vi "一体站流程平行样自动启动.vi"(11 "参数":T1) -> ()   [LabVIEW 2016, in "质控单元.lvlib"]
panel:
  out "枚举":enum16{"初始化", "采配水启动", "等待", "配水", "排水", "结束"}(ring)
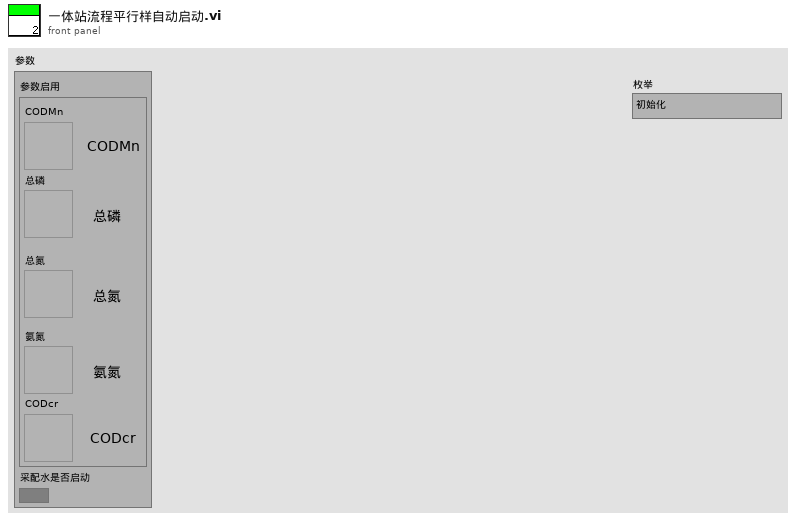
[diagram p1: front panel]
types:
  T1 = cluster{"参数启用":cluster{"CODMn":bool, "总磷":bool, "总氮":bool, "氨氮":bool, "CODcr":bool}, "采配水是否启动":bool}
  T2 = cluster{"命令":string, cluster{"starting address":u16, "holding register value":u16}}
  T3 = typedef "质控单元.lvlib/平行样测试流程.ctl" = enum16{"待机", "第一次水样测试启动", "第一次水样测试中", "第二次水样测试启动", "第二次水样测试中", "存储平行样测试数据", "结束"}
  T4 = cluster{"站号":u16, "量程切换":enum32{"H", "L", "AUTO"}, "控制命令":enum16{"启动测量", "标样核查", "零点核查", "跨度核查", "空白测试", "平行样测试", "加标回收", "空白校准", "标样校准", "初始化（清洗）", "停止测试", "仪器重启", "校时", "模式设置", "测量间隔设置"}, "模式设置":enum16{"待机", "连续模式", "周期模式", "定点模式", "受控模式", "手动模式"}, "测量间隔":u16}
  T5 = cluster{"时间标识":timestamp, "设备":string, "日志信息":string}
  T6 = enum16{"空闲", "水样测试", "标样核查", "零点核查", "跨度核查", "空白测试", "平行样测试", "加标回收", "空白校准", "标样校准", "初始化（清洗）"}
  T7 = cluster{"测量模式":enum16{"水样测量", "标样核查", "零点核查", "跨度核查", "空白测试", "加标回收", "平行样", "校零", "校标"}}
  T8 = cluster{"时间标识":timestamp, "设备":string, "日志信息":string, "流程参数":string}
  T9 = cluster{"R0":i16, "R1":i16, "R2":i16, "R3":i16, "R4":i16, "R5":i16, "R6":i16, "R7":i16, "R8":i16, "R9":i16, "R10":i16, "R11":i16, "R12":i16, "R13":i16, "R14":i16, "R15":i16, "R16":i16, "R17":i16, "R18":i16, "R19":i16, "R20":i16, "R21":i16, "R22":i16, "R23":i16, "R24":i16, "R25":i16, "R26":i16, "R27":i16, "R28":i16, "R29":i16, "R30":i16, "R31":i16, "R32":i16, "R33":i16, "R34":i16, "R35":i16, "R36":i16, "R37":i16, "R38":i16, "R39":i16, "R40":i16, "R41":i16, "R42":i16, "R43":i16, "R44":i16, "R45":i16, "R46":i16, "R47":i16, "R48":i16, "R49":i16, "R50":i16, "R51":i16, "R52":i16, "R53":i16, "R54":i16, "R55":i16, "R56":i16}
  T10 = cluster{"系统时间":timestamp, "工作状态":enum16{"空闲", "水样测试", "标样核查", "零点核查", "跨度核查", "空白测试", "平行样测试", "加标回收", "空白校准", "标样校准", "初始化（清洗）"}, "测量模式":enum16{"待机", "连续模式", "周期模式", "定点模式", "受控模式", "手动模式"}, "告警代码":enum16{"无告警", "缺试剂告警", "缺水样告警", "缺蒸馏水告警", "缺标液告警", "仪表漏液告警", "标定异常告警", "超量程告警", "加热异常", "低试剂预警", "超上限告警", "超下限告警", "仪表内部其他异常", "滴定异常告警", "电极异常告警", "量程切换告警", "参数设置告警", "PH电极电位异常", "电导率电极异常", "浊度光度异常", "溶解氧电极异常", "溶解氧光强异常", "温度异常告警", "PH异常告警", "溶解氧异常告警", "电导率异常告警", "浊度异常告警", "叶绿素异常告警", "藻密度异常告警", "蓝绿藻异常告警", "ORP异常告警", "氨氮异常告警", "清洁刷异常告警", "SD卡异常告警", "蓝牙异常告警", "Wifi异常告警", "流程异常告警"}, "故障代码":enum16{"无故障", "电机故障", "温度故障", "通讯故障", "滴定故障"}, "日志代码":u16, "软件版本":u16, "F0":sgl, "F1":sgl, "F2":sgl, "F3":sgl, "T":sgl, "H":sgl, "id":u16, "flowid":u16, "量程":u16, "总磷控温温度1":sgl, "营养盐控温温度2":sgl, "ADC":sgl}
  T11 = cluster{"因子编码":u32, "单位":u16, "标样参考值":sgl, "水样数据时间":timestamp, "水样实测值":sgl, "水样数据标识":string, "标样数据时间":timestamp, "标样实测值":sgl, "标样数据标识":string, "空白数据时间":timestamp, "空白实测值":sgl, "空白数据标识":string, "零点核查数据时间":timestamp, "零点核查实测值":sgl, "零点核查数据标识":string, "跨度核查数据时间":timestamp, "跨度核查实测值":sgl, "跨度核查数据标识":string, "加标回收数据时间":timestamp, "加标回收实测值":sgl, "加标回收数据标识":string, "平行样数据时间":timestamp, "平行样实测值":sgl, "平行样数据标识":string}
  T12 = cluster{"时间标识":timestamp, "参数":string, "数据类型":string, "第一次水样浓度值":sgl, "第二次水样测试时间":timestamp, "第二次水样浓度值":sgl}
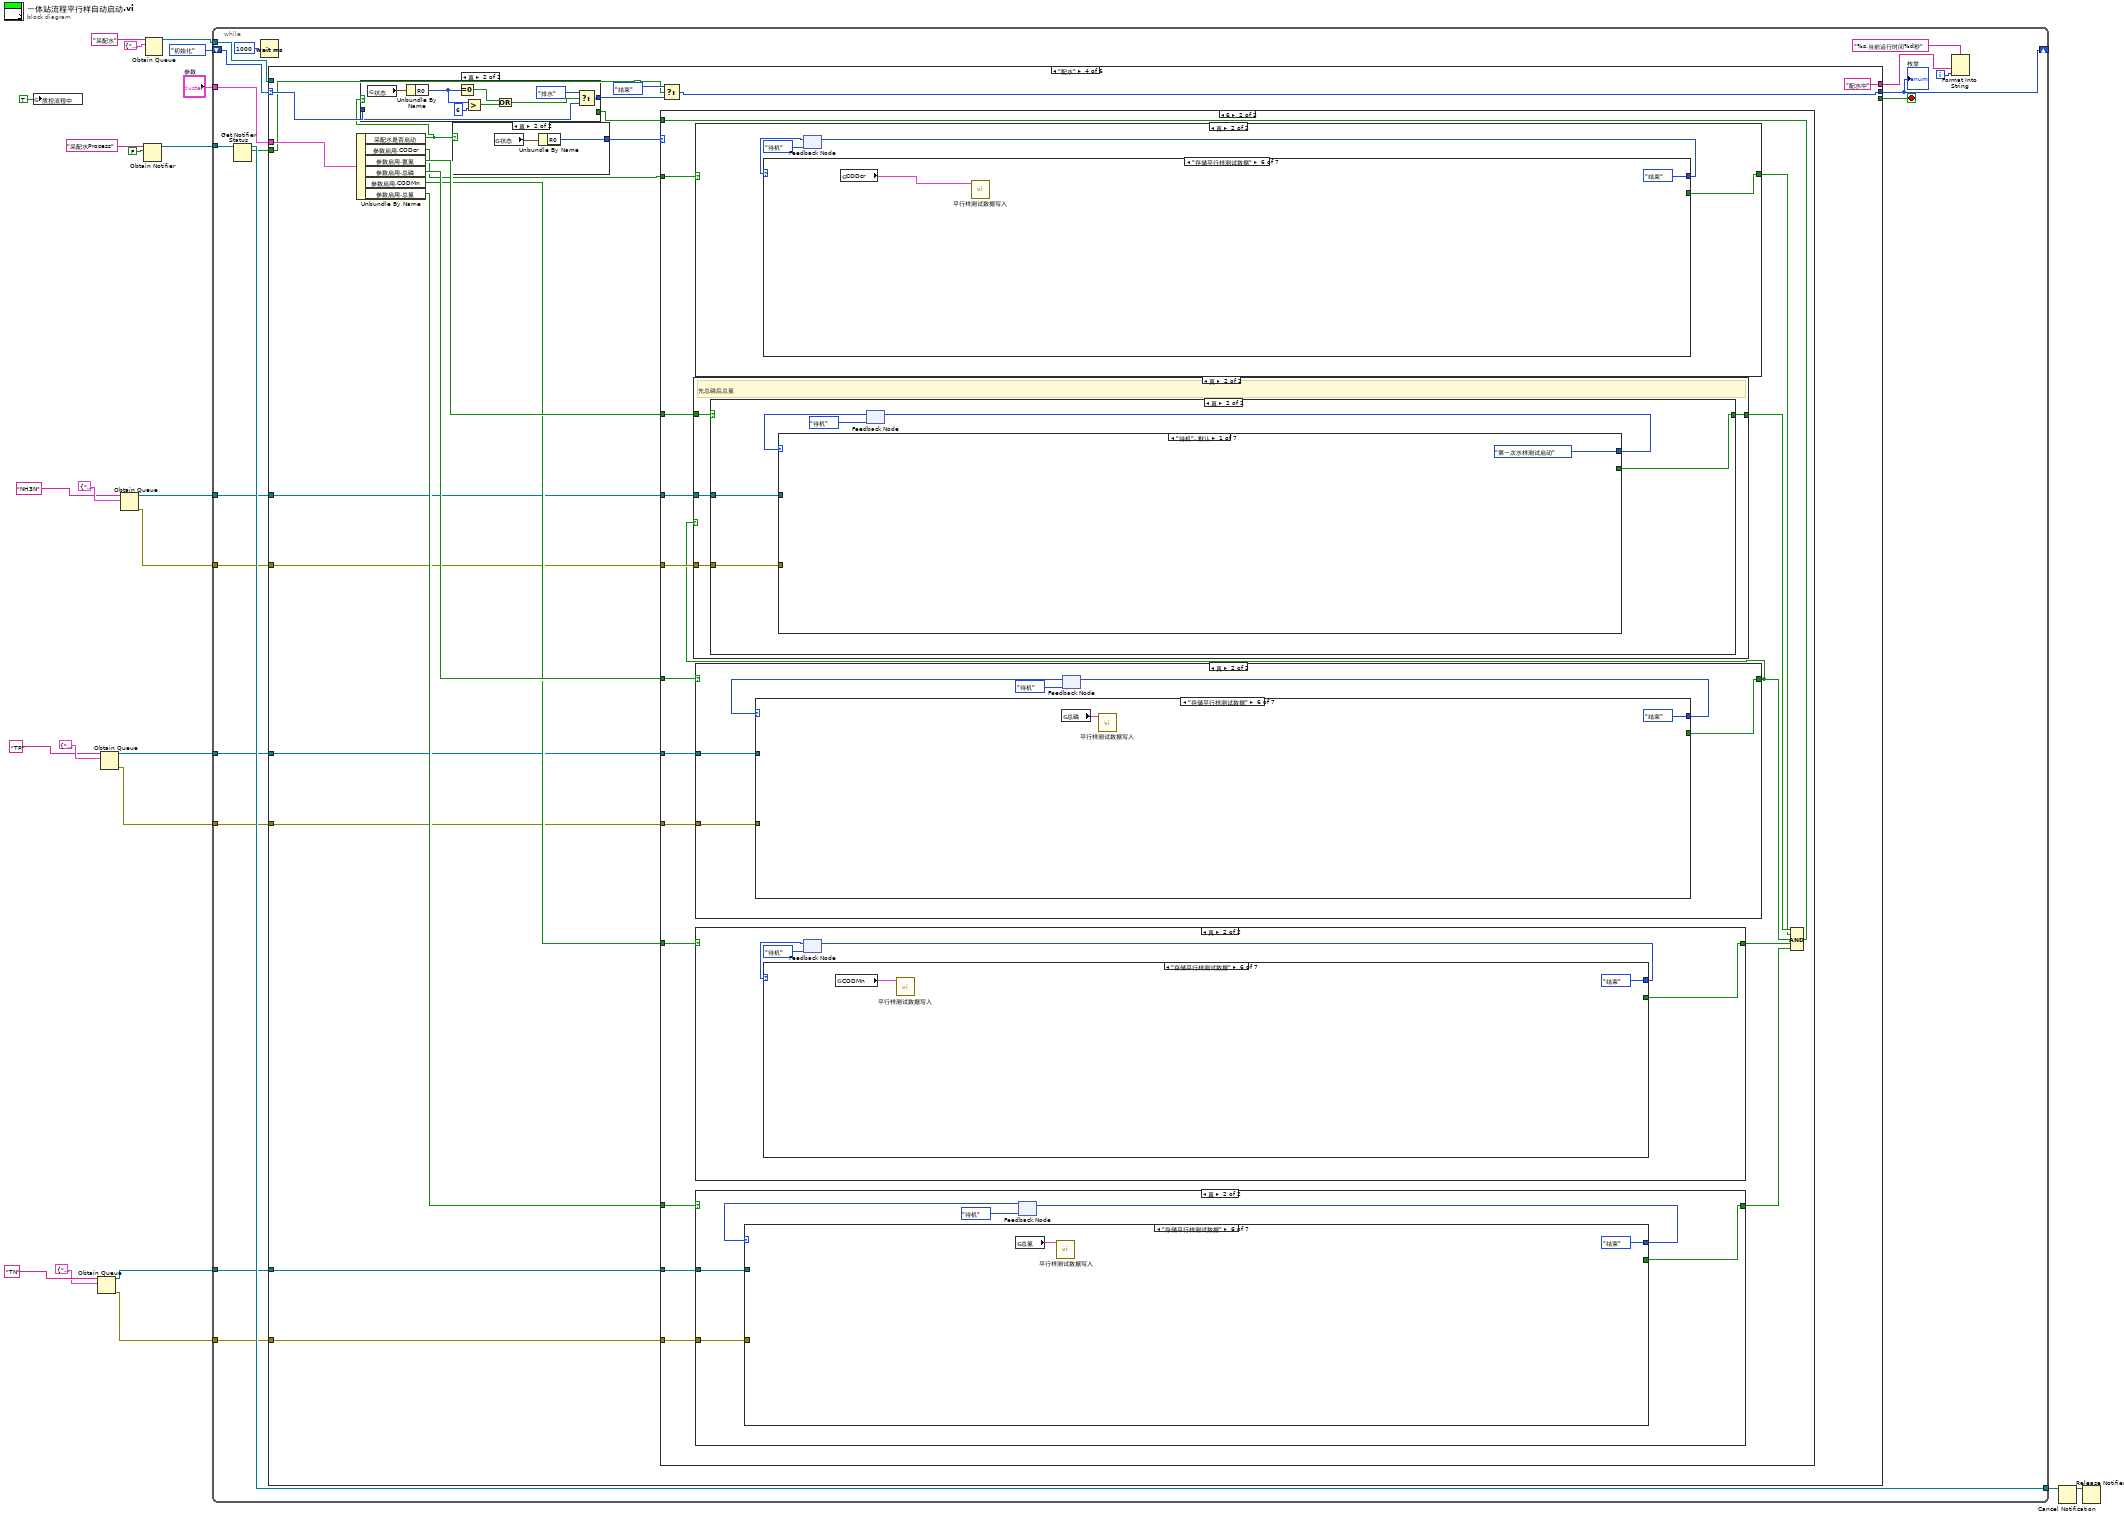
[diagram p0: block diagram]
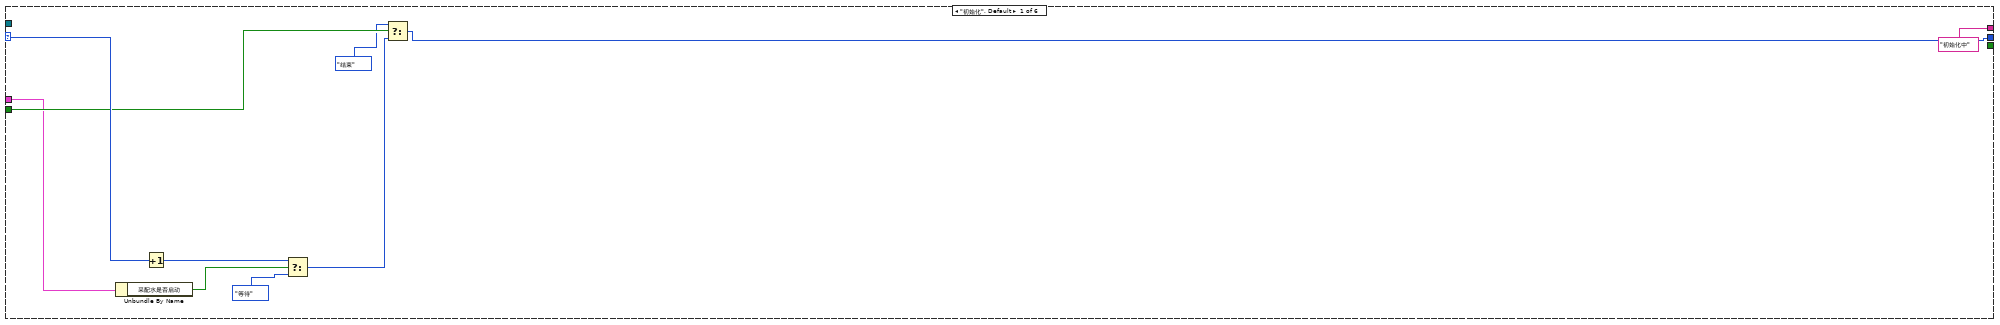
[diagram p2: hidden frame]
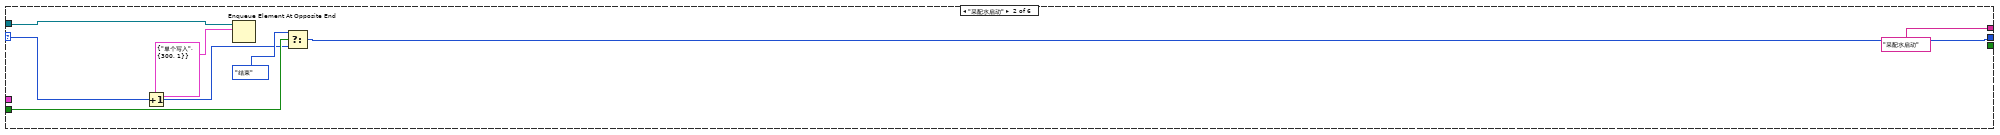
[diagram p3: hidden frame]
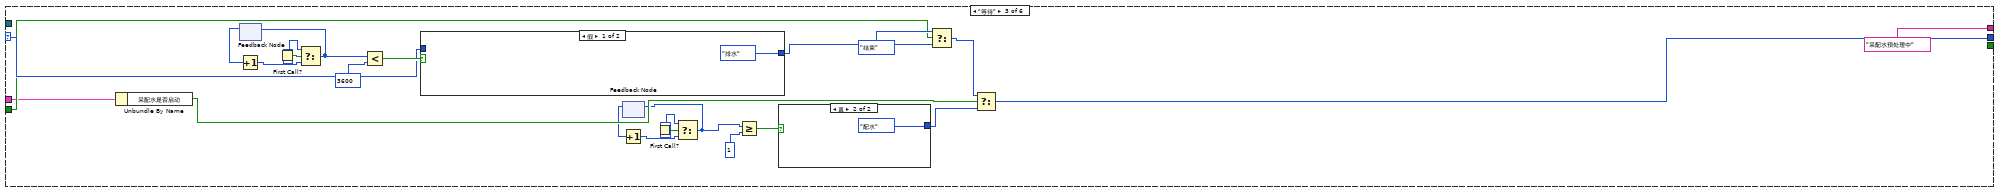
[diagram p4: hidden frame]
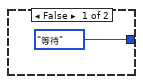
[diagram p5: hidden frame]
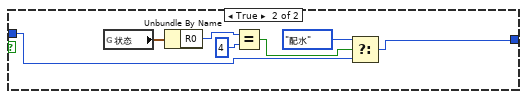
[diagram p6: hidden frame]
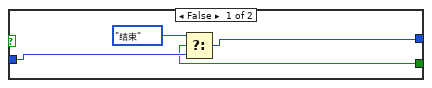
[diagram p7: hidden frame]
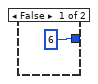
[diagram p8: hidden frame]
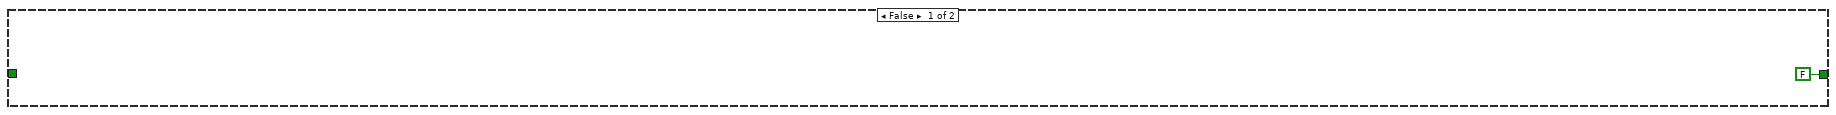
[diagram p10: hidden frame]
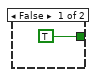
[diagram p11: hidden frame]
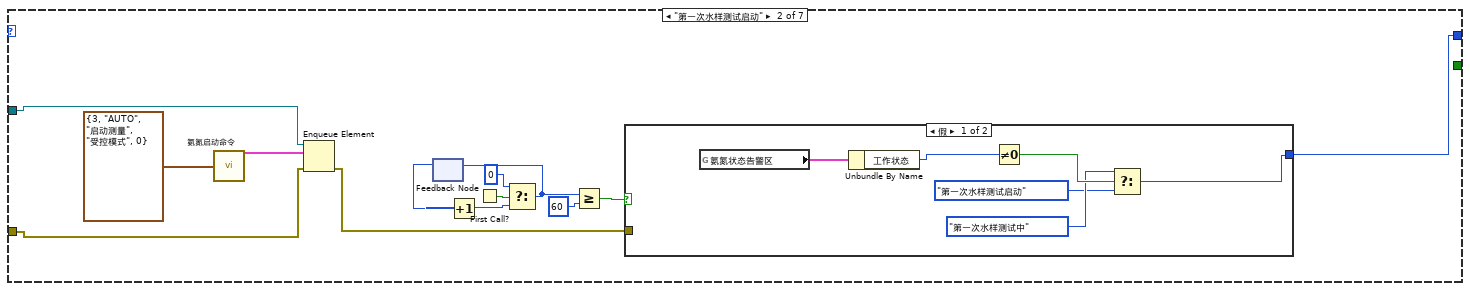
[diagram p12: hidden frame]
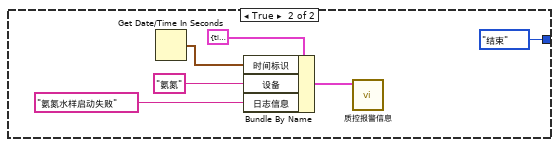
[diagram p13: hidden frame]
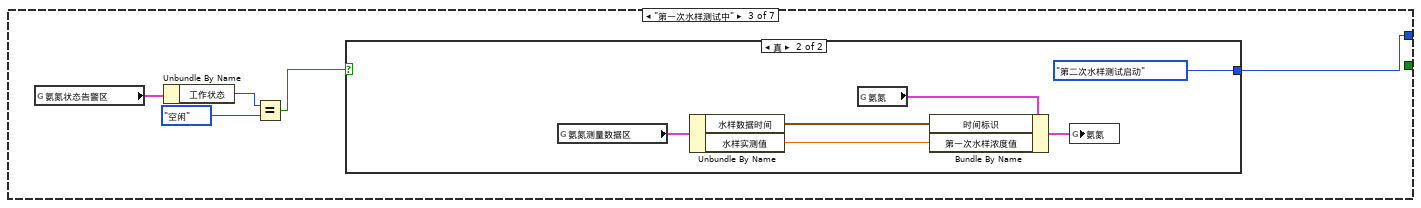
[diagram p14: hidden frame]
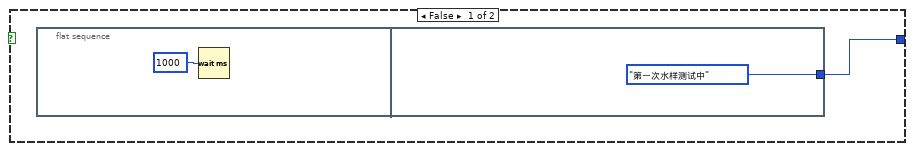
[diagram p15: hidden frame]
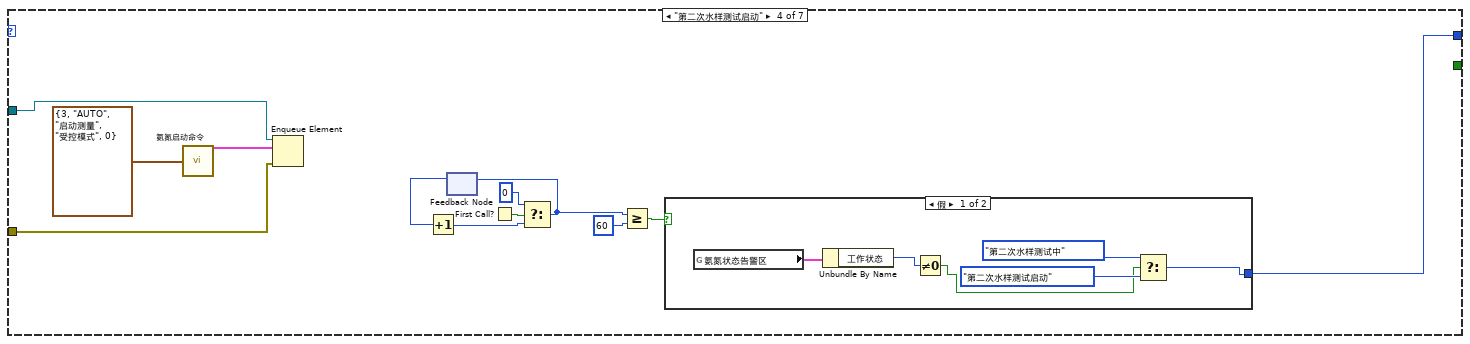
[diagram p16: hidden frame]
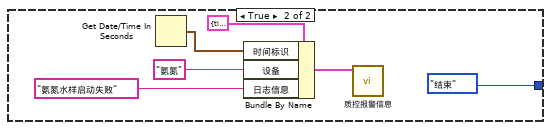
[diagram p17: hidden frame]
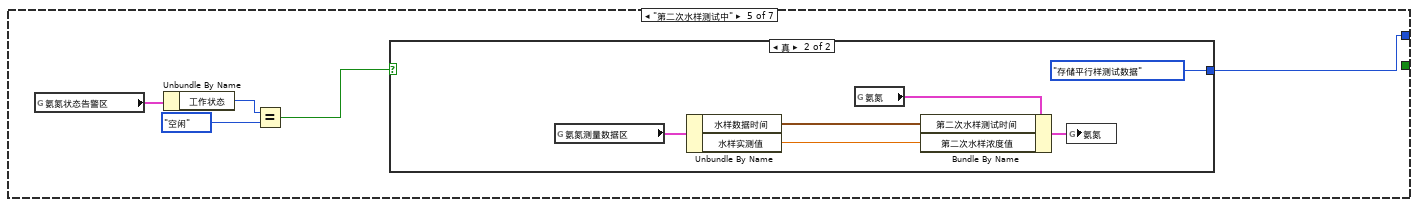
[diagram p18: hidden frame]
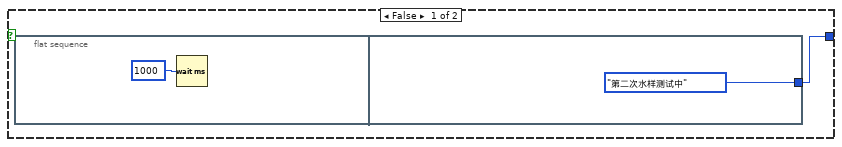
[diagram p19: hidden frame]
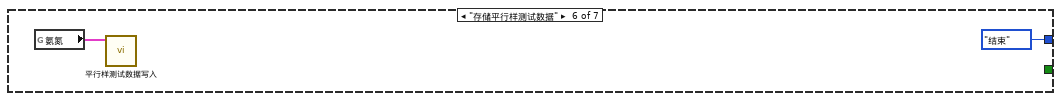
[diagram p20: hidden frame]
diagram:
  n1 = global write "质控测完标志全局 1.vi" "质控流程中"(TRUE ("质控流程中")) -> ()
  n2 = Obtain Queue(name (unnamed)="TN" ("名称（未命名）"), element data type=cluster{"命令":string, "data":variant} {"命令"="", "data"=variant}) -> (queue out=w3:refnum<queue>, error out=w2:errorcluster)  [unwired: 3 in, 1 out]
  n3 = Obtain Queue(name (unnamed)="TP" ("名称（未命名）"), element data type=cluster{"命令":string, "data":variant} {"命令"="", "data"=variant}) -> (queue out=w5:refnum<queue>, error out=w4:errorcluster)  [unwired: 3 in, 1 out]
  n4 = Obtain Queue(name (unnamed)="NH3N" ("名称（未命名）"), element data type=cluster{"命令":string, "data":variant} {"命令"="", "data"=variant}) -> (queue out=w7:refnum<queue>, error out=w6:errorcluster)  [unwired: 3 in, 1 out]
  n5 = Obtain Notifier(name (unnamed)="采配水Process" ("名称（未命名）"), notification data type=FALSE) -> (notifier out=w16:refnum<notifier>)  [unwired: 2 in, 2 out]
  n6 = Obtain Queue(name (unnamed)="采配水" ("名称（未命名）"), element data type=cluster{"命令":string, "数据":variant} {"命令"="", "数据"=variant}) -> (queue out=w21:refnum<queue>)  [unwired: 3 in, 2 out]
  n7 = while {
    tunnel: w21 -> [w41]
    shift-right: [w39] -> _
    shift-left: enum16{"初始化", "采配水启动", "等待", "配水", "排水", "结束"}."初始化" ("枚举") -> [w40]
    tunnel: "参数" -> [w37]
    tunnel: w16 -> [w36]
    tunnel: [w35] -> w15
    tunnel: w7 -> [w30]
    tunnel: w6 -> [w29]
    tunnel: w5 -> [w28]
    tunnel: w4 -> [w27]
    tunnel: w3 -> [w26]
    tunnel: w2 -> [w25]
    i -> [w32]
    stop <- w24 stop-if-true
    n8 = Get Notifier Status(notifier=w36) -> (notifier out=w35:refnum<notifier>, current notification=w31:bool)  [unwired: 1 in, 3 out]
    n9 = Wait (ms)(milliseconds to wait=u32 1000 ("等待时间（毫秒）")) -> ()  [unwired: 1 out]
    n10 = case shown="\"配水\"" w40 {
      selector: w40 -> [w51 w57 w81 w114 w596 w603]
      tunnel: w41 -> [_ w58 _ _ w597 _]
      tunnel: [w48 w52 w60 w111 w591 w602] -> w39
      tunnel: [_ _ _ _ _ TRUE] -> w24
      tunnel: w37 -> [w46 _ w71 w107 _ _]
      tunnel: ["初始化中" ("输入 1") "采配水启动" ("输入 1") "采配水预处理中" ("输入 1") "配水中" ("输入 1") "排水中" ("输入 1") "结束" ("输入 1")] -> w33
      tunnel: w31 -> [w49 w54 w73 w95 w593 _]
      tunnel: w30 -> [_ _ _ w102 _ _]
      tunnel: w29 -> [_ _ _ w101 _ _]
      tunnel: w28 -> [_ _ _ w100 _ _]
      tunnel: w27 -> [_ _ _ w99 _ _]
      tunnel: w26 -> [_ _ _ w98 _ _]
      tunnel: w25 -> [_ _ _ w97 _ _]
      frame "初始化", Default {
        n11 = Unbundle By Name(w46) -> ("采配水是否启动"=w45:bool)
        n12 = Increment(x=w51) -> (x+1=w44:enum16{"初始化", "采配水启动", "等待", "配水", "排水", "结束"})
        n13 = Select(t=w44, s=w45, f=enum16{"初始化", "采配水启动", "等待", "配水", "排水", "结束"}."等待") -> (s? t:f=w43:enum16{"初始化", "采配水启动", "等待", "配水", "排水", "结束"})
        n14 = Select(t=enum16{"初始化", "采配水启动", "等待", "配水", "排水", "结束"}."结束", s=w49, f=w43) -> (s? t:f=w48:enum16{"初始化", "采配水启动", "等待", "配水", "排水", "结束"})
      }
      frame "采配水启动" {
        n15 = Increment(x=w57) -> (x+1=w53:enum16{"初始化", "采配水启动", "等待", "配水", "排水", "结束"})
        n16 = Enqueue Element At Opposite End(queue=w58, element=T2 {"命令"="单个写入", {"starting address"=300, "holding register value"=1}} ("元素")) -> ()  [unwired: 2 in, 3 out]
        n17 = Select(t=enum16{"初始化", "采配水启动", "等待", "配水", "排水", "结束"}."结束", s=w54, f=w53) -> (s? t:f=w52:enum16{"初始化", "采配水启动", "等待", "配水", "排水", "结束"})
      }
      frame "等待" {
        n18 = Unbundle By Name(w71) -> ("采配水是否启动"=w70:bool)
        n19 = feedback #1() -> (w78:i32)  [unwired: 1 in]
        n20 = Increment(x=w78) -> (x+1=w77:i32)
        n21 = First Call?() -> (First Call?: T/F=w79:bool)
        n22 = Select(t=0, s=w79, f=w77) -> (s? t:f=w76:i32)
        n23 = feedback-in #1(w76) -> ()
        n24 = Less?(x=w76, y=3600) -> (x < y?=w82:bool)
        n25 = case shown="假" w82 {
          tunnel: w81 -> [_ w88]
          tunnel: [enum16{"初始化", "采配水启动", "等待", "配水", "排水", "结束"}."排水" ("枚举") w87] -> w72
          frame False {
          }
          frame True {
            n26 = global read "与采配水交互全局.vi" "状态"() -> (w93:T9)
            n27 = Unbundle By Name(w93) -> ("R0"=w92:i16)
            n28 = Equal?(x=w92, y=i16 4) -> (x = y?=w90:bool)
            n29 = Select(t=enum16{"初始化", "采配水启动", "等待", "配水", "排水", "结束"}."配水" ("枚举"), s=w90, f=w88) -> (s? t:f=w87:enum16{"初始化", "采配水启动", "等待", "配水", "排水", "结束"})
          }
        }
        n30 = feedback #2() -> (w66:i32)  [unwired: 1 in]
        n31 = Increment(x=w66) -> (x+1=w67:i32)
        n32 = First Call?() -> (First Call?: T/F=w65:bool)
        n33 = Select(t=0, s=w65, f=w67) -> (s? t:f=w68:i32)
        n34 = feedback-in #2(w68) -> ()
        n35 = Greater Or Equal?(x=w68, y=1) -> (x >= y?=w62:bool)
        n36 = case shown="真" w62 {
          tunnel: [enum16{"初始化", "采配水启动", "等待", "配水", "排水", "结束"}."等待" ("t") enum16{"初始化", "采配水启动", "等待", "配水", "排水", "结束"}."配水" ("t")] -> w61
          frame False {
          }
          frame True {
          }
        }
        n37 = Select(t=enum16{"初始化", "采配水启动", "等待", "配水", "排水", "结束"}."结束", s=w73, f=w72) -> (s? t:f=w69:enum16{"初始化", "采配水启动", "等待", "配水", "排水", "结束"})
        n38 = Select(t=w69, s=w70, f=w61) -> (s? t:f=w60:enum16{"初始化", "采配水启动", "等待", "配水", "排水", "结束"})
      }
      frame "配水" {
        n39 = Unbundle By Name(w107) -> ("采配水是否启动"=w96:bool, "参数启用.CODcr"=w106:bool, "参数启用.氨氮"=w110:bool, "参数启用.总磷"=w109:bool, "参数启用.CODMn"=w108:bool, "参数启用.总氮"=w105:bool)
        n40 = case shown="真" w96 {
          tunnel: [i16 6 ("R0") w129] -> w104
          frame False {
          }
          frame True {
            n41 = global read "与采配水交互全局.vi" "状态"() -> (w130:T9)
            n42 = Unbundle By Name(w130) -> ("R0"=w129:i16)
          }
        }
        n43 = case shown="6" w104 {
          tunnel: w110 -> [_ w147]
          tunnel: w109 -> [_ w146]
          tunnel: w108 -> [_ w144]
          tunnel: w106 -> [_ w143]
          tunnel: w105 -> [_ w140]
          tunnel: w102 -> [_ w138]
          tunnel: w101 -> [_ w137]
          tunnel: w100 -> [_ w136]
          tunnel: w99 -> [_ w135]
          tunnel: w98 -> [_ w134]
          tunnel: w97 -> [_ w133]
          tunnel: [_ w132] -> w94
          frame 0, Default {
          }
          frame 6 {
            n44 = case shown="真" w143 {
              tunnel: [TRUE w408] -> w142
              frame False {
              }
              frame True {
                n45 = feedback #3(平行样测试流程."待机") -> (w410:T3)
                n46 = case shown="\"存储平行样测试数据\"" w410 {
                  tunnel: [平行样测试流程."第一次水样测试启动" w422 w444 w464 w486 平行样测试流程."结束" 平行样测试流程."结束"] -> w409
                  tunnel: [_ _ _ _ _ _ TRUE] -> w408
                  frame "待机", Default {
                  }
                  frame "第一次水样测试启动" {
                    n47 = call "CODCr启动命令 (子VI).vi"("启动测量模式"=T7 {"测量模式"=enum."水样测量"}) -> ("错误输出"=w412:errorcluster)  [unwired: 10 in]
                    n48 = First Call?() -> (First Call?: T/F=w414:bool)
                    n49 = case shown="真" w414 {
                      frame False {
                      }
                      frame True {
                        n50 = Get Date/Time In Seconds() -> (seconds since 1Jan1904=w425:timestamp)
                        n51 = Bundle By Name(cluster=T8 {"时间标识"=timestamp(0 s since 1904-01-01), "设备"="", "日志信息"="", "流程参数"=""} ("data in"), "时间标识"=w425, "设备"="CODCr", "日志信息"="-->>CODCr启动水样") -> (w426:T8)
                        n52 = call "质控日志存储 (子VI).vi"("data in"=w426) -> ()  [unwired: 11 in]
                      }
                    }
                    n53 = feedback #4() -> (w418:i32)  [unwired: 1 in]
                    n54 = Increment(x=w418) -> (x+1=w419:i32)
                    n55 = First Call?() -> (First Call?: T/F=w417:bool)
                    n56 = Select(t=0, s=w417, f=w419) -> (s? t:f=w420:i32)
                    n57 = feedback-in #4(w420) -> ()
                    n58 = Greater Or Equal?(x=w420, y=60) -> (x >= y?=w415:bool)
                    n59 = case shown="假" w415 {
                      tunnel: [w432 平行样测试流程."结束"] -> w422
                      tunnel: w412 -> [_ _]
                      frame False {
                        n60 = global read "与CODCr交互全局.vi" "CODCr状态告警区"() -> (w429:T10)
                        n61 = Unbundle By Name(w429) -> ("工作状态"=w428:T6)
                        n62 = Not Equal To 0?(x=w428) -> (x != 0?=w433:bool)
                        n63 = Select(t=平行样测试流程."第一次水样测试中", s=w433, f=平行样测试流程."第一次水样测试启动") -> (s? t:f=w432:T3)
                      }
                      frame True {
                        n64 = Get Date/Time In Seconds() -> (seconds since 1Jan1904=w436:timestamp)
                        n65 = Bundle By Name(cluster=T5 {"时间标识"=timestamp(0 s since 1904-01-01), "设备"="", "日志信息"=""} ("data in"), "时间标识"=w436, "设备"="CODCr", "日志信息"="CODCr水样启动失败") -> (w434:T5)
                        n66 = call "质控报警信息.vi"("data in"=w434) -> ()  [unwired: 11 in]
                      }
                    }
                  }
                  frame "第一次水样测试中" {
                    n67 = global read "与CODCr交互全局.vi" "CODCr状态告警区"() -> (w443:T10)
                    n68 = Unbundle By Name(w443) -> ("工作状态"=w440:T6)
                    n69 = Equal?(x=w440, y=T6."空闲" ("工作状态")) -> (x = y?=w442:bool)
                    n70 = case shown="真" w442 {
                      tunnel: [w445 平行样测试流程."第二次水样测试启动"] -> w444
                      frame False {
                        n71 = flat-sequence {
                          tunnel: [平行样测试流程."第一次水样测试中"] -> w445
                          frame #0 {
                            n72 = Wait (ms)(milliseconds to wait=u32 1000 ("等待时间（毫秒）")) -> ()  [unwired: 1 out]
                          }
                          frame #1 {
                          }
                        }
                      }
                      frame True {
                        n73 = global read "与CODCr交互全局.vi" "CODCr测量数据区"() -> (w450:T11)
                        n74 = Unbundle By Name(w450) -> ("水样数据时间"=w449:timestamp, "水样实测值"=w448:sgl)
                        n75 = global read "平行样测试全局变量.vi" "CODcr"() -> (w452:T12)
                        n76 = Bundle By Name(cluster=w452, "时间标识"=w449, "第一次水样浓度值"=w448) -> (w451:T12)
                        n77 = global write "平行样测试全局变量.vi" "CODcr"(w451) -> ()
                      }
                    }
                  }
                  frame "第二次水样测试启动" {
                    n78 = call "CODCr启动命令 (子VI).vi"("启动测量模式"=T7 {"测量模式"=enum."水样测量"}) -> ("错误输出"=w454:errorcluster)  [unwired: 10 in]
                    n79 = First Call?() -> (First Call?: T/F=w456:bool)
                    n80 = case shown="真" w456 {
                      frame False {
                      }
                      frame True {
                        n81 = Get Date/Time In Seconds() -> (seconds since 1Jan1904=w467:timestamp)
                        n82 = Bundle By Name(cluster=T8 {"时间标识"=timestamp(0 s since 1904-01-01), "设备"="", "日志信息"="", "流程参数"=""} ("data in"), "时间标识"=w467, "设备"="CODCr", "日志信息"="-->>CODCr启动水样") -> (w468:T8)
                        n83 = call "质控日志存储 (子VI).vi"("data in"=w468) -> ()  [unwired: 11 in]
                      }
                    }
                    n84 = First Call?() -> (First Call?: T/F=w459:bool)
                    n85 = feedback #5() -> (w460:i32)  [unwired: 1 in]
                    n86 = Increment(x=w460) -> (x+1=w461:i32)
                    n87 = Select(t=0, s=w459, f=w461) -> (s? t:f=w462:i32)
                    n88 = feedback-in #5(w462) -> ()
                    n89 = Greater Or Equal?(x=w462, y=60) -> (x >= y?=w457:bool)
                    n90 = case shown="假" w457 {
                      tunnel: [w474 平行样测试流程."结束"] -> w464
                      tunnel: w454 -> [_ _]
                      frame False {
                        n91 = global read "与CODCr交互全局.vi" "CODCr状态告警区"() -> (w471:T10)
                        n92 = Unbundle By Name(w471) -> ("工作状态"=w470:T6)
                        n93 = Not Equal To 0?(x=w470) -> (x != 0?=w475:bool)
                        n94 = Select(t=平行样测试流程."第二次水样测试中", s=w475, f=平行样测试流程."第二次水样测试启动") -> (s? t:f=w474:T3)
                      }
                      frame True {
                        n95 = Get Date/Time In Seconds() -> (seconds since 1Jan1904=w478:timestamp)
                        n96 = Bundle By Name(cluster=T5 {"时间标识"=timestamp(0 s since 1904-01-01), "设备"="", "日志信息"=""} ("data in"), "时间标识"=w478, "设备"="CODCr", "日志信息"="CODCr启动失败") -> (w476:T5)
                        n97 = call "质控报警信息.vi"("data in"=w476) -> ()  [unwired: 11 in]
                      }
                    }
                  }
                  frame "第二次水样测试中" {
                    n98 = global read "与CODCr交互全局.vi" "CODCr状态告警区"() -> (w485:T10)
                    n99 = Unbundle By Name(w485) -> ("工作状态"=w482:T6)
                    n100 = Equal?(x=w482, y=T6."空闲" ("工作状态")) -> (x = y?=w484:bool)
                    n101 = case shown="假" w484 {
                      tunnel: [w487 平行样测试流程."存储平行样测试数据"] -> w486
                      frame False {
                        n102 = flat-sequence {
                          tunnel: [平行样测试流程."第二次水样测试中"] -> w487
                          frame #0 {
                            n103 = Wait (ms)(milliseconds to wait=u32 1000 ("等待时间（毫秒）")) -> ()  [unwired: 1 out]
                          }
                          frame #1 {
                          }
                        }
                      }
                      frame True {
                        n104 = global read "与CODCr交互全局.vi" "CODCr测量数据区"() -> (w492:T11)
                        n105 = Unbundle By Name(w492) -> ("水样数据时间"=w491:timestamp, "水样实测值"=w490:sgl)
                        n106 = global read "平行样测试全局变量.vi" "CODcr"() -> (w494:T12)
                        n107 = Bundle By Name(cluster=w494, "第二次水样测试时间"=w491, "第二次水样浓度值"=w490) -> (w493:T12)
                        n108 = global write "平行样测试全局变量.vi" "CODcr"(w493) -> ()
                      }
                    }
                  }
                  frame "存储平行样测试数据" {
                    n109 = global read "平行样测试全局变量.vi" "CODcr"() -> (w496:T12)
                    n110 = call "平行样测试数据写入.vi"("data"=w496) -> ()  [unwired: 10 in, 1 out]
                  }
                  frame "结束" {
                    n111 = First Call?() -> (First Call?: T/F=w499:bool)
                    n112 = case shown="真" w499 {
                      frame False {
                      }
                      frame True {
                        (unwired) "-->>CODCr停止" ("日志信息")
                        (unwired) "CODCr" ("设备")
                        n113 = call "质控日志存储 (子VI).vi"() -> ()  [unwired: 12 in]
                      }
                    }
                  }
                }
                n114 = feedback-in #3(w409) -> ()
              }
            }
            n115 = case shown="真" w146 {
              tunnel: [TRUE w505] -> w131
              tunnel: w136 -> [_ w503]
              tunnel: w135 -> [_ w502]
              frame False {
              }
              frame True {
                n116 = feedback #6(平行样测试流程."待机") -> (w507:T3)
                n117 = case shown="\"存储平行样测试数据\"" w507 {
                  tunnel: [平行样测试流程."第一次水样测试启动" w509 w538 w548 w573 平行样测试流程."结束" 平行样测试流程."结束"] -> w506
                  tunnel: [_ _ _ _ _ _ TRUE] -> w505
                  tunnel: w503 -> [_ w521 _ w550 _ _ _]
                  tunnel: w502 -> [_ w520 _ w549 _ _ _]
                  frame "待机", Default {
                  }
                  frame "第一次水样测试启动" {
                    n118 = call "总磷启动命令.vi"("参数"=T4 {"站号"=1, "量程切换"=enum."AUTO", "控制命令"=enum."启动测量", "模式设置"=enum."受控模式", "测量间隔"=0}) -> ("启动命令"=w519:cluster{"命令":string, "data":variant})  [unwired: 10 in]
                    n119 = Enqueue Element(queue=w521, element=w519, error in (no error)=w520) -> (error out=w510:errorcluster)  [unwired: 1 in, 2 out]
                    n120 = feedback #7() -> (w514:i32)  [unwired: 1 in]
                    n121 = Increment(x=w514) -> (x+1=w513:i32)
                    n122 = First Call?() -> (First Call?: T/F=w515:bool)
                    n123 = Select(t=0, s=w515, f=w513) -> (s? t:f=w512:i32)
                    n124 = feedback-in #7(w512) -> ()
                    n125 = Greater Or Equal?(x=w512, y=60) -> (x >= y?=w517:bool)
                    n126 = case shown="假" w517 {
                      tunnel: [w526 平行样测试流程."结束"] -> w509
                      tunnel: w510 -> [_ _]
                      frame False {
                        n127 = global read "与总磷交互全局.vi" "总磷状态告警区"() -> (w522:T10)
                        n128 = Unbundle By Name(w522) -> ("工作状态"=w523:T6)
                        n129 = Not Equal To 0?(x=w523) -> (x != 0?=w527:bool)
                        n130 = Select(t=平行样测试流程."第一次水样测试中", s=w527, f=平行样测试流程."第一次水样测试启动") -> (s? t:f=w526:T3)
                      }
                      frame True {
                        n131 = Get Date/Time In Seconds() -> (seconds since 1Jan1904=w530:timestamp)
                        n132 = Bundle By Name(cluster=T5 {"时间标识"=timestamp(0 s since 1904-01-01), "设备"="", "日志信息"=""} ("data in"), "时间标识"=w530, "设备"="总磷", "日志信息"="总磷水样启动失败") -> (w528:T5)
                        n133 = call "质控报警信息.vi"("data in"=w528) -> ()  [unwired: 11 in]
                      }
                    }
                  }
                  frame "第一次水样测试中" {
                    n134 = global read "与总磷交互全局.vi" "总磷状态告警区"() -> (w534:T10)
                    n135 = Unbundle By Name(w534) -> ("工作状态"=w537:T6)
                    n136 = Equal?(x=w537, y=T6."空闲" ("工作状态")) -> (x = y?=w535:bool)
                    n137 = case shown="真" w535 {
                      tunnel: [w539 平行样测试流程."第二次水样测试启动"] -> w538
                      frame False {
                        n138 = flat-sequence {
                          tunnel: [平行样测试流程."第一次水样测试中"] -> w539
                          frame #0 {
                            n139 = Wait (ms)(milliseconds to wait=u32 1000 ("等待时间（毫秒）")) -> ()  [unwired: 1 out]
                          }
                          frame #1 {
                          }
                        }
                      }
                      frame True {
                        n140 = global read "与总磷交互全局.vi" "总磷测量数据区"() -> (w542:T11)
                        n141 = Unbundle By Name(w542) -> ("水样数据时间"=w545:timestamp, "水样实测值"=w546:sgl)
                        n142 = global read "平行样测试全局变量.vi" "总磷"() -> (w543:T12)
                        n143 = Bundle By Name(cluster=w543, "时间标识"=w545, "第一次水样浓度值"=w546) -> (w544:T12)
                        n144 = global write "平行样测试全局变量.vi" "总磷"(w544) -> ()
                      }
                    }
                  }
                  frame "第二次水样测试启动" {
                    n145 = call "总磷启动命令.vi"("参数"=T4 {"站号"=1, "量程切换"=enum."AUTO", "控制命令"=enum."启动测量", "模式设置"=enum."受控模式", "测量间隔"=0}) -> ("启动命令"=w560:cluster{"命令":string, "data":variant})  [unwired: 10 in]
                    n146 = Enqueue Element(queue=w550, element=w560, error in (no error)=w549) -> (error out=w551:errorcluster)  [unwired: 1 in, 2 out]
                    n147 = feedback #8() -> (w555:i32)  [unwired: 1 in]
                    n148 = Increment(x=w555) -> (x+1=w554:i32)
                    n149 = First Call?() -> (First Call?: T/F=w556:bool)
                    n150 = Select(t=0, s=w556, f=w554) -> (s? t:f=w553:i32)
                    n151 = feedback-in #8(w553) -> ()
                    n152 = Greater Or Equal?(x=w553, y=60) -> (x >= y?=w558:bool)
                    n153 = case shown="假" w558 {
                      tunnel: [w565 平行样测试流程."结束"] -> w548
                      tunnel: w551 -> [_ _]
                      frame False {
                        n154 = global read "与总磷交互全局.vi" "总磷状态告警区"() -> (w561:T10)
                        n155 = Unbundle By Name(w561) -> ("工作状态"=w562:T6)
                        n156 = Not Equal To 0?(x=w562) -> (x != 0?=w566:bool)
                        n157 = Select(t=平行样测试流程."第二次水样测试中", s=w566, f=平行样测试流程."第二次水样测试启动") -> (s? t:f=w565:T3)
                      }
                      frame True {
                        n158 = Get Date/Time In Seconds() -> (seconds since 1Jan1904=w569:timestamp)
                        n159 = Bundle By Name(cluster=T5 {"时间标识"=timestamp(0 s since 1904-01-01), "设备"="", "日志信息"=""} ("data in"), "时间标识"=w569, "设备"="总磷", "日志信息"="总磷水样启动失败") -> (w567:T5)
                        n160 = call "质控报警信息.vi"("data in"=w567) -> ()  [unwired: 11 in]
                      }
                    }
                  }
                  frame "第二次水样测试中" {
                    n161 = global read "与总磷交互全局.vi" "总磷状态告警区"() -> (w574:T10)
                    n162 = Unbundle By Name(w574) -> ("工作状态"=w577:T6)
                    n163 = Equal?(x=w577, y=T6."空闲" ("工作状态")) -> (x = y?=w575:bool)
                    n164 = case shown="真" w575 {
                      tunnel: [w578 平行样测试流程."存储平行样测试数据"] -> w573
                      frame False {
                        n165 = flat-sequence {
                          tunnel: [平行样测试流程."第二次水样测试中"] -> w578
                          frame #0 {
                            n166 = Wait (ms)(milliseconds to wait=u32 1000 ("等待时间（毫秒）")) -> ()  [unwired: 1 out]
                          }
                          frame #1 {
                          }
                        }
                      }
                      frame True {
                        n167 = global read "与总磷交互全局.vi" "总磷测量数据区"() -> (w581:T11)
                        n168 = Unbundle By Name(w581) -> ("水样数据时间"=w584:timestamp, "水样实测值"=w585:sgl)
                        n169 = global read "平行样测试全局变量.vi" "总磷"() -> (w582:T12)
                        n170 = Bundle By Name(cluster=w582, "第二次水样测试时间"=w584, "第二次水样浓度值"=w585) -> (w583:T12)
                        n171 = global write "平行样测试全局变量.vi" "总磷"(w583) -> ()
                      }
                    }
                  }
                  frame "存储平行样测试数据" {
                    n172 = global read "平行样测试全局变量.vi" "总磷"() -> (w587:T12)
                    n173 = call "平行样测试数据写入.vi"("data"=w587) -> ()  [unwired: 10 in, 1 out]
                  }
                  frame "结束" {
                  }
                }
                n174 = feedback-in #6(w506) -> ()
              }
            }
            n175 = case shown="真" w131 {
              tunnel: w147 -> [_ w152]
              tunnel: [FALSE w151] -> w145
              tunnel: w138 -> [_ w150]
              tunnel: w137 -> [_ w149]
              frame False {
              }
              frame True {
                # "先总磷后总氮"
                n176 = case shown="真" w152 {
                  tunnel: [TRUE w156] -> w151
                  tunnel: w150 -> [_ w155]
                  tunnel: w149 -> [_ w154]
                  frame False {
                  }
                  frame True {
                    n177 = feedback #9(平行样测试流程."待机") -> (w158:T3)
                    n178 = case shown="\"待机\", 默认" w158 {
                      tunnel: [平行样测试流程."第一次水样测试启动" w161 w190 w204 w228 平行样测试流程."结束" 平行样测试流程."结束"] -> w157
                      tunnel: [_ _ _ _ _ _ TRUE] -> w156
                      tunnel: w155 -> [_ w171 _ w201 _ _ _]
                      tunnel: w154 -> [_ w170 _ w200 _ _ _]
                      frame "待机", Default {
                      }
                      frame "第一次水样测试启动" {
                        n179 = call "氨氮启动命令.vi"("参数"=T4 {"站号"=3, "量程切换"=enum."AUTO", "控制命令"=enum."启动测量", "模式设置"=enum."受控模式", "测量间隔"=0}) -> ("启动命令"=w173:cluster{"命令":string, "data":variant})  [unwired: 10 in]
                        n180 = Enqueue Element(queue=w171, element=w173, error in (no error)=w170) -> (error out=w162:errorcluster)  [unwired: 1 in, 2 out]
                        n181 = feedback #10() -> (w166:i32)  [unwired: 1 in]
                        n182 = Increment(x=w166) -> (x+1=w167:i32)
                        n183 = First Call?() -> (First Call?: T/F=w165:bool)
                        n184 = Select(t=0, s=w165, f=w167) -> (s? t:f=w168:i32)
                        n185 = feedback-in #10(w168) -> ()
                        n186 = Greater Or Equal?(x=w168, y=60) -> (x >= y?=w163:bool)
                        n187 = case shown="假" w163 {
                          tunnel: [w178 平行样测试流程."结束"] -> w161
                          tunnel: w162 -> [_ _]
                          frame False {
                            n188 = global read "与氨氮交互全局.vi" "氨氮状态告警区"() -> (w174:T10)
                            n189 = Unbundle By Name(w174) -> ("工作状态"=w175:T6)
                            n190 = Not Equal To 0?(x=w175) -> (x != 0?=w179:bool)
                            n191 = Select(t=平行样测试流程."第一次水样测试中", s=w179, f=平行样测试流程."第一次水样测试启动") -> (s? t:f=w178:T3)
                          }
                          frame True {
                            n192 = Get Date/Time In Seconds() -> (seconds since 1Jan1904=w182:timestamp)
                            n193 = Bundle By Name(cluster=T5 {"时间标识"=timestamp(0 s since 1904-01-01), "设备"="", "日志信息"=""} ("data in"), "时间标识"=w182, "设备"="氨氮", "日志信息"="氨氮水样启动失败") -> (w180:T5)
                            n194 = call "质控报警信息.vi"("data in"=w180) -> ()  [unwired: 11 in]
                          }
                        }
                      }
                      frame "第一次水样测试中" {
                        n195 = global read "与氨氮交互全局.vi" "氨氮状态告警区"() -> (w189:T10)
                        n196 = Unbundle By Name(w189) -> ("工作状态"=w187:T6)
                        n197 = Equal?(x=w187, y=T6."空闲" ("工作状态")) -> (x = y?=w186:bool)
                        n198 = case shown="真" w186 {
                          tunnel: [w191 平行样测试流程."第二次水样测试启动"] -> w190
                          frame False {
                            n199 = flat-sequence {
                              tunnel: [平行样测试流程."第一次水样测试中"] -> w191
                              frame #0 {
                                n200 = Wait (ms)(milliseconds to wait=u32 1000 ("等待时间（毫秒）")) -> ()  [unwired: 1 out]
                              }
                              frame #1 {
                              }
                            }
                          }
                          frame True {
                            n201 = global read "与氨氮交互全局.vi" "氨氮测量数据区"() -> (w196:T11)
                            n202 = Unbundle By Name(w196) -> ("水样数据时间"=w195:timestamp, "水样实测值"=w194:sgl)
                            n203 = global read "平行样测试全局变量.vi" "氨氮"() -> (w198:T12)
                            n204 = Bundle By Name(cluster=w198, "时间标识"=w195, "第一次水样浓度值"=w194) -> (w197:T12)
                            n205 = global write "平行样测试全局变量.vi" "氨氮"(w197) -> ()
                          }
                        }
                      }
                      frame "第二次水样测试启动" {
                        n206 = call "氨氮启动命令.vi"("参数"=T4 {"站号"=3, "量程切换"=enum."AUTO", "控制命令"=enum."启动测量", "模式设置"=enum."受控模式", "测量间隔"=0}) -> ("启动命令"=w203:cluster{"命令":string, "data":variant})  [unwired: 10 in]
                        n207 = Enqueue Element(queue=w201, element=w203, error in (no error)=w200) -> ()  [unwired: 1 in, 3 out]
                        n208 = feedback #11() -> (w208:i32)  [unwired: 1 in]
                        n209 = Increment(x=w208) -> (x+1=w209:i32)
                        n210 = First Call?() -> (First Call?: T/F=w207:bool)
                        n211 = Select(t=0, s=w207, f=w209) -> (s? t:f=w210:i32)
                        n212 = feedback-in #11(w210) -> ()
                        n213 = Greater Or Equal?(x=w210, y=60) -> (x >= y?=w205:bool)
                        n214 = case shown="假" w205 {
                          tunnel: [w214 平行样测试流程."结束"] -> w204
                          frame False {
                            n215 = global read "与氨氮交互全局.vi" "氨氮状态告警区"() -> (w217:T10)
                            n216 = Unbundle By Name(w217) -> ("工作状态"=w213:T6)
                            n217 = Not Equal To 0?(x=w213) -> (x != 0?=w212:bool)
                            n218 = Select(t=平行样测试流程."第二次水样测试中", s=w212, f=平行样测试流程."第二次水样测试启动") -> (s? t:f=w214:T3)
                          }
                          frame True {
                            n219 = Get Date/Time In Seconds() -> (seconds since 1Jan1904=w220:timestamp)
                            n220 = Bundle By Name(cluster=T5 {"时间标识"=timestamp(0 s since 1904-01-01), "设备"="", "日志信息"=""} ("data in"), "时间标识"=w220, "设备"="氨氮", "日志信息"="氨氮水样启动失败") -> (w219:T5)
                            n221 = call "质控报警信息.vi"("data in"=w219) -> ()  [unwired: 11 in]
                          }
                        }
                      }
                      frame "第二次水样测试中" {
                        n222 = global read "与氨氮交互全局.vi" "氨氮状态告警区"() -> (w227:T10)
                        n223 = Unbundle By Name(w227) -> ("工作状态"=w225:T6)
                        n224 = Equal?(x=w225, y=T6."空闲" ("工作状态")) -> (x = y?=w224:bool)
                        n225 = case shown="真" w224 {
                          tunnel: [w229 平行样测试流程."存储平行样测试数据"] -> w228
                          frame False {
                            n226 = flat-sequence {
                              tunnel: [平行样测试流程."第二次水样测试中"] -> w229
                              frame #0 {
                                n227 = Wait (ms)(milliseconds to wait=u32 1000 ("等待时间（毫秒）")) -> ()  [unwired: 1 out]
                              }
                              frame #1 {
                              }
                            }
                          }
                          frame True {
                            n228 = global read "与氨氮交互全局.vi" "氨氮测量数据区"() -> (w234:T11)
                            n229 = Unbundle By Name(w234) -> ("水样数据时间"=w233:timestamp, "水样实测值"=w232:sgl)
                            n230 = global read "平行样测试全局变量.vi" "氨氮"() -> (w236:T12)
                            n231 = Bundle By Name(cluster=w236, "第二次水样测试时间"=w233, "第二次水样浓度值"=w232) -> (w235:T12)
                            n232 = global write "平行样测试全局变量.vi" "氨氮"(w235) -> ()
                          }
                        }
                      }
                      frame "存储平行样测试数据" {
                        n233 = global read "平行样测试全局变量.vi" "氨氮"() -> (w238:T12)
                        n234 = call "平行样测试数据写入.vi"("data"=w238) -> ()  [unwired: 10 in, 1 out]
                      }
                      frame "结束" {
                      }
                    }
                    n235 = feedback-in #9(w157) -> ()
                  }
                }
              }
            }
            n236 = case shown="真" w144 {
              tunnel: [TRUE w334] -> w141
              frame False {
              }
              frame True {
                n237 = feedback #12(平行样测试流程."待机") -> (w336:T3)
                n238 = case shown="\"存储平行样测试数据\"" w336 {
                  tunnel: [平行样测试流程."第一次水样测试启动" w347 w361 w379 w393 平行样测试流程."结束" 平行样测试流程."结束"] -> w335
                  tunnel: [_ _ _ _ _ _ TRUE] -> w334
                  frame "待机", Default {
                  }
                  frame "第一次水样测试启动" {
                    n239 = feedback #13() -> (w343:i32)  [unwired: 1 in]
                    n240 = Increment(x=w343) -> (x+1=w344:i32)
                    n241 = call "CODMn启动命令 (子VI).vi"("启动测量模式"=T7 {"测量模式"=enum."水样测量"}) -> ("错误输出"=w338:errorcluster)  [unwired: 10 in]
                    n242 = First Call?() -> (First Call?: T/F=w342:bool)
                    n243 = Select(t=0, s=w342, f=w344) -> (s? t:f=w345:i32)
                    n244 = feedback-in #13(w345) -> ()
                    n245 = Greater Or Equal?(x=w345, y=60) -> (x >= y?=w340:bool)
                    n246 = case shown="真" w340 {
                      tunnel: [w351 平行样测试流程."结束"] -> w347
                      tunnel: w338 -> [_ _]
                      frame False {
                        n247 = global read "与CODMn交互全局.vi" "多列列表框"() -> (w350:i32)
                        n248 = Not Equal To 0?(x=w350) -> (x != 0?=w352:bool)
                        n249 = Select(t=平行样测试流程."第一次水样测试中", s=w352, f=平行样测试流程."第一次水样测试启动") -> (s? t:f=w351:T3)
                      }
                      frame True {
                        n250 = Get Date/Time In Seconds() -> (seconds since 1Jan1904=w355:timestamp)
                        n251 = Bundle By Name(cluster=T5 {"时间标识"=timestamp(0 s since 1904-01-01), "设备"="", "日志信息"=""} ("data in"), "时间标识"=w355, "设备"="CODMn", "日志信息"="CODMn启动失败") -> (w353:T5)
                        n252 = call "质控报警信息.vi"("data in"=w353) -> ()  [unwired: 11 in]
                      }
                    }
                  }
                  frame "第一次水样测试中" {
                    n253 = global read "与CODMn交互全局.vi" "多列列表框"() -> (w360:i32)
                    n254 = Equal To 0?(x=w360) -> (x = 0?=w359:bool)
                    n255 = case shown="假" w359 {
                      tunnel: [w362 平行样测试流程."第二次水样测试启动"] -> w361
                      frame False {
                        n256 = flat-sequence {
                          tunnel: [平行样测试流程."第一次水样测试中"] -> w362
                          frame #0 {
                            n257 = Wait (ms)(milliseconds to wait=u32 1000 ("等待时间（毫秒）")) -> ()  [unwired: 1 out]
                          }
                          frame #1 {
                          }
                        }
                      }
                      frame True {
                        n258 = global read "与CODMn交互全局.vi" "COD浓度（mg/L)"() -> (w365:dbl)
                        n259 = global read "与CODMn交互全局.vi" "水样启动时间"() -> (w366:timestamp)
                        n260 = global read "平行样测试全局变量.vi" "CODMn"() -> (w368:T12)
                        n261 = Bundle By Name(cluster=w368, "时间标识"=w366, "第一次水样浓度值"=w365) -> (w367:T12)
                        n262 = global write "平行样测试全局变量.vi" "CODMn"(w367) -> ()
                      }
                    }
                  }
                  frame "第二次水样测试启动" {
                    n263 = feedback #14() -> (w375:i32)  [unwired: 1 in]
                    n264 = Increment(x=w375) -> (x+1=w376:i32)
                    n265 = First Call?() -> (First Call?: T/F=w374:bool)
                    n266 = call "CODMn启动命令 (子VI).vi"("启动测量模式"=T7 {"测量模式"=enum."水样测量"}) -> ("错误输出"=w370:errorcluster)  [unwired: 10 in]
                    n267 = Select(t=0, s=w374, f=w376) -> (s? t:f=w377:i32)
                    n268 = feedback-in #14(w377) -> ()
                    n269 = Greater Or Equal?(x=w377, y=60) -> (x >= y?=w372:bool)
                    n270 = case shown="真" w372 {
                      tunnel: [w383 平行样测试流程."结束"] -> w379
                      tunnel: w370 -> [_ _]
                      frame False {
                        n271 = global read "与CODMn交互全局.vi" "多列列表框"() -> (w382:i32)
                        n272 = Not Equal To 0?(x=w382) -> (x != 0?=w384:bool)
                        n273 = Select(t=平行样测试流程."第二次水样测试中", s=w384, f=平行样测试流程."第二次水样测试启动") -> (s? t:f=w383:T3)
                      }
                      frame True {
                        n274 = Get Date/Time In Seconds() -> (seconds since 1Jan1904=w387:timestamp)
                        n275 = Bundle By Name(cluster=T5 {"时间标识"=timestamp(0 s since 1904-01-01), "设备"="", "日志信息"=""} ("data in"), "时间标识"=w387, "设备"="CODMn", "日志信息"="CODMn启动失败") -> (w385:T5)
                        n276 = call "质控报警信息.vi"("data in"=w385) -> ()  [unwired: 11 in]
                      }
                    }
                  }
                  frame "第二次水样测试中" {
                    n277 = global read "与CODMn交互全局.vi" "多列列表框"() -> (w392:i32)
                    n278 = Equal To 0?(x=w392) -> (x = 0?=w391:bool)
                    n279 = case shown="真" w391 {
                      tunnel: [w394 平行样测试流程."存储平行样测试数据"] -> w393
                      frame False {
                        n280 = flat-sequence {
                          tunnel: [平行样测试流程."第二次水样测试中"] -> w394
                          frame #0 {
                            n281 = Wait (ms)(milliseconds to wait=u32 1000 ("等待时间（毫秒）")) -> ()  [unwired: 1 out]
                          }
                          frame #1 {
                          }
                        }
                      }
                      frame True {
                        n282 = global read "与CODMn交互全局.vi" "COD浓度（mg/L)"() -> (w397:dbl)
                        n283 = global read "与CODMn交互全局.vi" "水样启动时间"() -> (w398:timestamp)
                        n284 = global read "平行样测试全局变量.vi" "CODMn"() -> (w400:T12)
                        n285 = Bundle By Name(cluster=w400, "时间标识"=w398, "第一次水样浓度值"=w397) -> (w399:T12)
                        n286 = global write "平行样测试全局变量.vi" "CODMn"(w399) -> ()
                      }
                    }
                  }
                  frame "存储平行样测试数据" {
                    n287 = global read "平行样测试全局变量.vi" "CODMn"() -> (w402:T12)
                    n288 = call "平行样测试数据写入.vi"("data"=w402) -> ()  [unwired: 10 in, 1 out]
                  }
                  frame "结束" {
                  }
                }
                n289 = feedback-in #12(w335) -> ()
              }
            }
            n290 = case shown="真" w140 {
              tunnel: [TRUE w246] -> w139
              tunnel: w134 -> [_ w244]
              tunnel: w133 -> [_ w243]
              frame False {
              }
              frame True {
                n291 = feedback #15(平行样测试流程."待机") -> (w248:T3)
                n292 = case shown="\"存储平行样测试数据\"" w248 {
                  tunnel: [平行样测试流程."第一次水样测试启动" w250 w276 w289 w314 平行样测试流程."结束" 平行样测试流程."结束"] -> w247
                  tunnel: [_ _ _ _ _ _ TRUE] -> w246
                  tunnel: w244 -> [_ w254 _ w291 _ _ _]
                  tunnel: w243 -> [_ w253 _ w290 _ _ _]
                  frame "待机", Default {
                  }
                  frame "第一次水样测试启动" {
                    n293 = call "总氮启动命令.vi"("参数"=T4 {"站号"=2, "量程切换"=enum."AUTO", "控制命令"=enum."启动测量", "模式设置"=enum."待机", "测量间隔"=0}) -> ("启动命令"=w252:cluster{"命令":string, "data":variant})  [unwired: 10 in]
                    n294 = Enqueue Element(queue=w254, element=w252, error in (no error)=w253) -> (error out=w255:errorcluster)  [unwired: 1 in, 2 out]
                    n295 = feedback #16() -> (w259:i32)  [unwired: 1 in]
                    n296 = Increment(x=w259) -> (x+1=w258:i32)
                    n297 = First Call?() -> (First Call?: T/F=w260:bool)
                    n298 = Select(t=0, s=w260, f=w258) -> (s? t:f=w257:i32)
                    n299 = feedback-in #16(w257) -> ()
                    n300 = Greater Or Equal?(x=w257, y=60) -> (x >= y?=w262:bool)
                    n301 = case shown="假" w262 {
                      tunnel: [w267 平行样测试流程."结束"] -> w250
                      tunnel: w255 -> [_ _]
                      frame False {
                        n302 = global read "与总氮交互全局.vi" "总氮状态告警区"() -> (w263:T10)
                        n303 = Unbundle By Name(w263) -> ("工作状态"=w264:T6)
                        n304 = Not Equal To 0?(x=w264) -> (x != 0?=w268:bool)
                        n305 = Select(t=平行样测试流程."第一次水样测试中", s=w268, f=平行样测试流程."第一次水样测试启动") -> (s? t:f=w267:T3)
                      }
                      frame True {
                        n306 = Get Date/Time In Seconds() -> (seconds since 1Jan1904=w271:timestamp)
                        n307 = Bundle By Name(cluster=T5 {"时间标识"=timestamp(0 s since 1904-01-01), "设备"="", "日志信息"=""} ("data in"), "时间标识"=w271, "设备"="总氮", "日志信息"="总氮水样启动失败") -> (w269:T5)
                        n308 = call "质控报警信息.vi"("data in"=w269) -> ()  [unwired: 11 in]
                      }
                    }
                  }
                  frame "第一次水样测试中" {
                    n309 = global read "与总氮交互全局.vi" "总氮状态告警区"() -> (w275:T10)
                    n310 = Unbundle By Name(w275) -> ("工作状态"=w279:T6)
                    n311 = Equal?(x=w279, y=T6."空闲" ("工作状态")) -> (x = y?=w277:bool)
                    n312 = case shown="真" w277 {
                      tunnel: [w280 平行样测试流程."第二次水样测试启动"] -> w276
                      frame False {
                        n313 = flat-sequence {
                          tunnel: [平行样测试流程."第一次水样测试中"] -> w280
                          frame #0 {
                            n314 = Wait (ms)(milliseconds to wait=u32 1000 ("等待时间（毫秒）")) -> ()  [unwired: 1 out]
                          }
                          frame #1 {
                          }
                        }
                      }
                      frame True {
                        n315 = global read "与总氮交互全局.vi" "总氮测量数据区"() -> (w283:T11)
                        n316 = Unbundle By Name(w283) -> ("水样数据时间"=w286:timestamp, "水样实测值"=w287:sgl)
                        n317 = global read "平行样测试全局变量.vi" "总氮"() -> (w284:T12)
                        n318 = Bundle By Name(cluster=w284, "时间标识"=w286, "第一次水样浓度值"=w287) -> (w285:T12)
                        n319 = global write "平行样测试全局变量.vi" "总氮"(w285) -> ()
                      }
                    }
                  }
                  frame "第二次水样测试启动" {
                    n320 = call "总氮启动命令.vi"("参数"=T4 {"站号"=2, "量程切换"=enum."AUTO", "控制命令"=enum."启动测量", "模式设置"=enum."待机", "测量间隔"=0}) -> ("启动命令"=w293:cluster{"命令":string, "data":variant})  [unwired: 10 in]
                    n321 = Enqueue Element(queue=w291, element=w293, error in (no error)=w290) -> (error out=w294:errorcluster)  [unwired: 1 in, 2 out]
                    n322 = feedback #17() -> (w298:i32)  [unwired: 1 in]
                    n323 = Increment(x=w298) -> (x+1=w297:i32)
                    n324 = First Call?() -> (First Call?: T/F=w299:bool)
                    n325 = Select(t=0, s=w299, f=w297) -> (s? t:f=w296:i32)
                    n326 = feedback-in #17(w296) -> ()
                    n327 = Greater Or Equal?(x=w296, y=60) -> (x >= y?=w301:bool)
                    n328 = case shown="假" w301 {
                      tunnel: [w306 平行样测试流程."结束"] -> w289
                      tunnel: w294 -> [_ _]
                      frame False {
                        n329 = global read "与总氮交互全局.vi" "总氮状态告警区"() -> (w302:T10)
                        n330 = Unbundle By Name(w302) -> ("工作状态"=w303:T6)
                        n331 = Not Equal To 0?(x=w303) -> (x != 0?=w307:bool)
                        n332 = Select(t=平行样测试流程."第二次水样测试中", s=w307, f=平行样测试流程."第二次水样测试启动") -> (s? t:f=w306:T3)
                      }
                      frame True {
                        n333 = Get Date/Time In Seconds() -> (seconds since 1Jan1904=w310:timestamp)
                        n334 = Bundle By Name(cluster=T5 {"时间标识"=timestamp(0 s since 1904-01-01), "设备"="", "日志信息"=""} ("data in"), "时间标识"=w310, "设备"="总氮", "日志信息"="总氮水样启动失败") -> (w308:T5)
                        n335 = call "质控报警信息.vi"("data in"=w308) -> ()  [unwired: 11 in]
                      }
                    }
                  }
                  frame "第二次水样测试中" {
                    n336 = global read "与总氮交互全局.vi" "总氮状态告警区"() -> (w315:T10)
                    n337 = Unbundle By Name(w315) -> ("工作状态"=w318:T6)
                    n338 = Equal?(x=w318, y=T6."空闲" ("工作状态")) -> (x = y?=w316:bool)
                    n339 = case shown="真" w316 {
                      tunnel: [w319 平行样测试流程."存储平行样测试数据"] -> w314
                      frame False {
                        n340 = flat-sequence {
                          tunnel: [平行样测试流程."第二次水样测试中"] -> w319
                          frame #0 {
                            n341 = Wait (ms)(milliseconds to wait=u32 1000 ("等待时间（毫秒）")) -> ()  [unwired: 1 out]
                          }
                          frame #1 {
                          }
                        }
                      }
                      frame True {
                        n342 = global read "与总氮交互全局.vi" "总氮测量数据区"() -> (w322:T11)
                        n343 = Unbundle By Name(w322) -> ("水样数据时间"=w325:timestamp, "水样实测值"=w326:sgl)
                        n344 = global read "平行样测试全局变量.vi" "总氮"() -> (w323:T12)
                        n345 = Bundle By Name(cluster=w323, "第二次水样测试时间"=w325, "第二次水样浓度值"=w326) -> (w324:T12)
                        n346 = global write "平行样测试全局变量.vi" "总氮"(w324) -> ()
                      }
                    }
                  }
                  frame "存储平行样测试数据" {
                    n347 = global read "平行样测试全局变量.vi" "总氮"() -> (w328:T12)
                    n348 = call "平行样测试数据写入.vi"("data"=w328) -> ()  [unwired: 10 in, 1 out]
                  }
                  frame "结束" {
                  }
                }
                n349 = feedback-in #15(w247) -> ()
              }
            }
            n350 = Compound Arithmetic op=AND ("复合运算")(w145, w142, w131, w141, w139) -> (w132:bool)
          }
        }
        n351 = case shown="真" w96 {
          tunnel: w114 -> [w117 w126]
          tunnel: [w116 w125] -> w112
          tunnel: w94 -> [w115 _]
          frame False {
            n352 = Select(t=enum16{"初始化", "采配水启动", "等待", "配水", "排水", "结束"}."结束" ("枚举"), s=w115, f=w117) -> (s? t:f=w116:enum16{"初始化", "采配水启动", "等待", "配水", "排水", "结束"})
          }
          frame True {
            n353 = global read "与采配水交互全局.vi" "状态"() -> (w124:T9)
            n354 = Unbundle By Name(w124) -> ("R0"=w123:i16)
            n355 = Equal To 0?(x=w123) -> (x = 0?=w120:bool)
            n356 = Greater?(x=w123, y=i16 6) -> (0:w121:bool)
            n357 = Or(x=w120, y=w121) -> (x .or. y?=w119:bool)
            n358 = Select(t=enum16{"初始化", "采配水启动", "等待", "配水", "排水", "结束"}."排水" ("枚举"), s=w119, f=w126) -> (s? t:f=w125:enum16{"初始化", "采配水启动", "等待", "配水", "排水", "结束"})
          }
        }
        n359 = Select(t=enum16{"初始化", "采配水启动", "等待", "配水", "排水", "结束"}."结束", s=w95, f=w112) -> (s? t:f=w111:enum16{"初始化", "采配水启动", "等待", "配水", "排水", "结束"})
      }
      frame "排水" {
        n360 = Increment(x=w596) -> (x+1=w592:enum16{"初始化", "采配水启动", "等待", "配水", "排水", "结束"})
        n361 = Enqueue Element At Opposite End(queue=w597, element=T2 {"命令"="单个写入", {"starting address"=303, "holding register value"=1}} ("元素")) -> ()  [unwired: 2 in, 3 out]
        n362 = Select(t=enum16{"初始化", "采配水启动", "等待", "配水", "排水", "结束"}."结束", s=w593, f=w592) -> (s? t:f=w591:enum16{"初始化", "采配水启动", "等待", "配水", "排水", "结束"})
      }
      frame "结束" {
        n363 = Increment(x=w603) -> (x+1=w602:enum16{"初始化", "采配水启动", "等待", "配水", "排水", "结束"})
        n364 = global write "质控测完标志全局 1.vi" "质控流程中"(FALSE ("质控流程中")) -> ()
      }
    }
    "枚举" <- w39
    n365 = Format Into String(format string="%s,当前运行时间%d秒" ("格式字符串"), w33, w32) -> ()  [unwired: 2 in, 2 out]
  }
  n366 = Cancel Notification(0:w15) -> (8:w14:refnum<notifier>)  [unwired: 1 in, 2 out]
  n367 = Release Notifier(notifier=w14) -> ()  [unwired: 2 in, 3 out]
